vi "Queue Loop.vi"(11 "Queue jettl in":refnum<class "Queue jettl.lvclass">) -> (3 "Queue jettl out":refnum<class "Queue jettl.lvclass">)   [LabVIEW 2021, in "jettl.lvlib" / "Queue jettl.lvclass"]
uses:
  Queue jettl.lvclass
  C:/git/jettl/src/jettl/jettl/jettl.lvclass
  Msg Strategy/Msg Strategy.lvclass
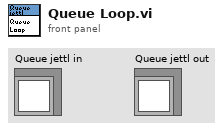
[diagram p1: front panel]
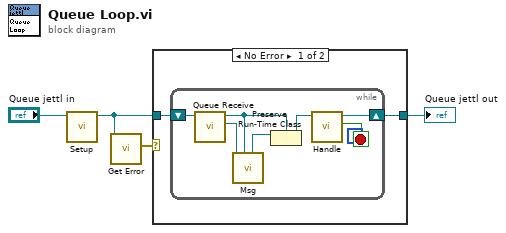
[diagram p0: block diagram]
diagram:
  n1 = call-dynamic "Setup.vi"("Setup in"="Queue jettl in") -> ("Setup out"=w3:refnum<class "Queue jettl.lvclass">)  [unwired: 10 in]
  n2 = call-dynamic "Get Error.vi"("jettl in"=w3) -> ("Error"=w4:errorcluster)  [unwired: 10 in]
  n3 = case shown="No Error" w4 {
    tunnel: [w6 w14] -> w1
    tunnel: w3 -> [w5 w14]
    frame No Error {
      n4 = while "Queue Loop" {
        shift-right: [w13] -> w6
        shift-left: w5 -> [w12]
        stop <- w10 stop-if-true
        n5 = call-dynamic "Queue Receive.vi"("Queue jettl in"=w12) -> ("Msg Strategy"=w11:refnum<class "Msg Strategy.lvclass">, "Queue jettl out"=w9:refnum<class "Queue jettl.lvclass">)  [unwired: 9 in]
        n6 = call-dynamic "Msg.vi"("jettl in"=w9, "Msg Strategy in"=w11) -> ("jettl out"=w7:refnum<class "jettl.lvclass">)  [unwired: 9 in]
        n7 = Preserve Run-Time Class(object in=w7, 2:w9) -> (object out=w8:refnum<class "Queue jettl.lvclass">)  [unwired: 1 in, 1 out]
        n8 = call-dynamic "Handle.vi"("jettl in"=w8) -> ("Destroy?"=w10:bool, "jettl out"=w13:refnum<class "Queue jettl.lvclass">)  [unwired: 9 in]
      }
    }
    frame Error {
    }
  }
  "Queue jettl out" <- w1
